vi "RandomNumPan.vi"(8 "error in (no error)":errorcluster caption="entrée d'erreur (pas d'erreur)", 11 "Tools.lvclass":refnum<class "Tools.lvclass">) -> (0 "error out":errorcluster caption="sortie d'erreur", 3 "Tools.lvclass Out":refnum<class "Tools.lvclass">)   [LabVIEW 2019, in "Tools.lvclass"]
uses:
  Tools.lvclass
  C:/Programmes Labview/LabScanV1A/DevicesClass/BaseDevice/BaseDevice.lvclass
  BaseDevice/Accessor/GetClassEvent.vi
panel:
  in  "Acq":bool
  in  "MainProgQ":refnum<queue>
  in  "MainProgQEvent":refnum<user-event>
  out "MultiplierOut":dbl=1.0
  out "OffsetOut":dbl
  out "Random Number":dbl
  in  "Multiplier":dbl=1.0
  in  "Offset":dbl
  in  "Stop":bool
  in  "MiseAJour":bool
  out "Init Program":bool
  # "Out = Random Number(0-1) x Mult. +Offset"
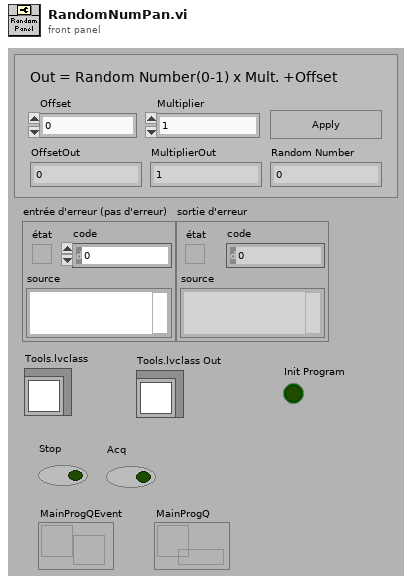
[diagram p1: front panel]
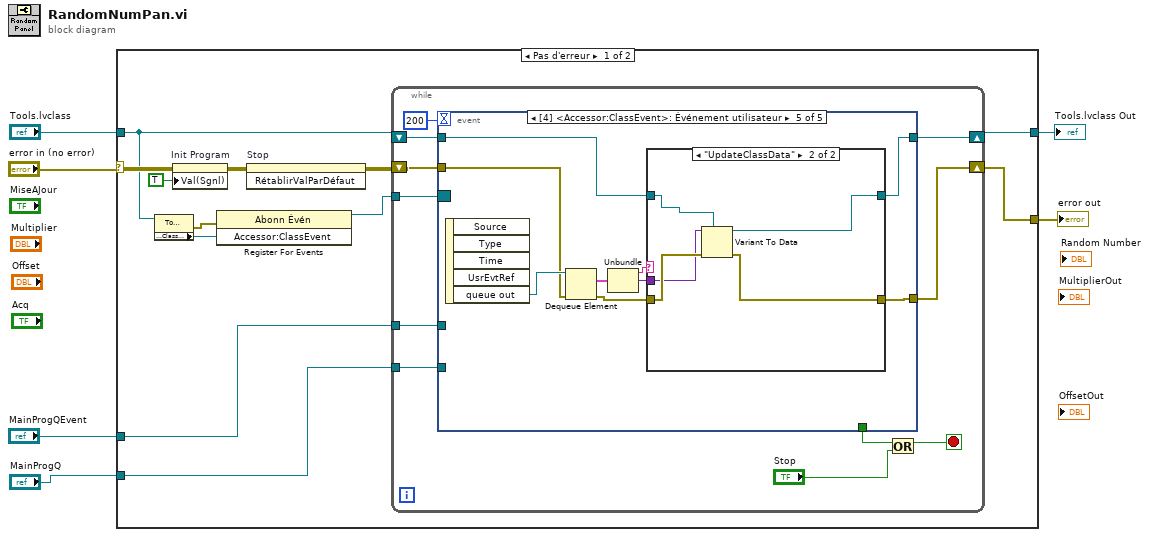
[diagram p0: block diagram]
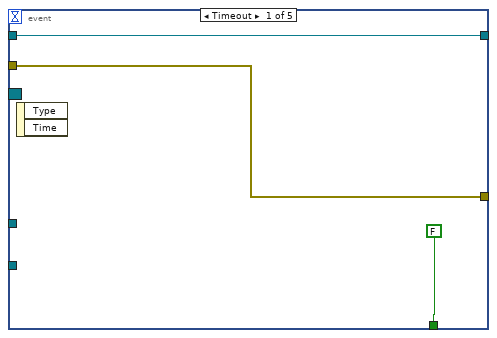
[diagram p2: hidden frame]
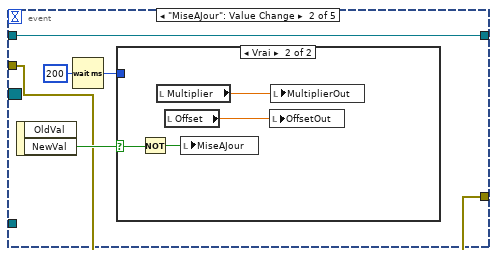
[diagram p3: hidden frame]
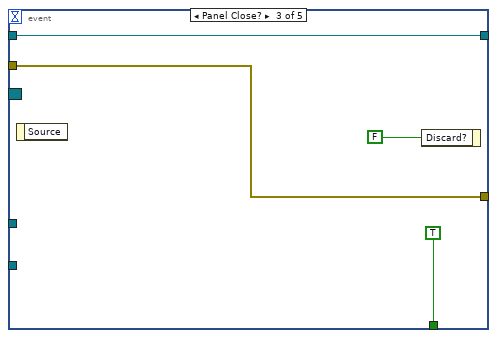
[diagram p5: hidden frame]
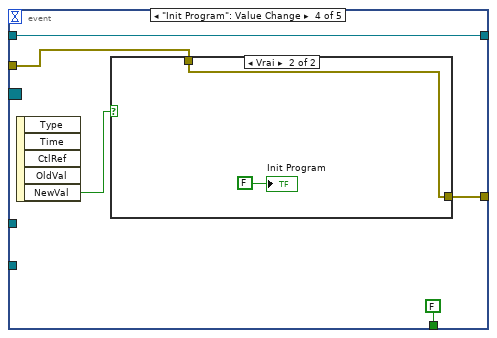
[diagram p6: hidden frame]
diagram:
  n1 = case shown="Pas d'erreur" "error in (no error)" {
    selector: "error in (no error)" -> [w15 w71]
    tunnel: [w18 w71] -> w5
    tunnel: "Tools.lvclass" -> [w8 w70]
    tunnel: [w16 w70] -> w3
    tunnel: "MainProgQEvent" -> [w12 _]
    tunnel: "MainProgQ" -> [w11 _]
    frame No Error {
      n2 = property class="Tools.lvclass"(reference=w8) -> (error out=w10:errorcluster, "Accessor:ClassEvent"=w9:refnum<user-event>)  [unwired: 1 in, 1 out]
      n3 = property on="Init Program" class="Bool (strict)"(error in=w15, "Val(Sgnl)"=TRUE ("Valeur (Signalisation)")) -> (error out=w14:errorcluster)  [unwired: 1 in, 1 out]
      n4 = register-events(error in=w10, w9) -> (reference out=w7:refnum<event-registration>)  [unwired: 1 in, 1 out]
      n5 = invoke on="Stop" class="Bool (strict)" method="RétablirValParDéfaut"(error in=w14) -> (error out=w13:errorcluster)  [unwired: 2 in, 2 out]
      n6 = while {
        shift-right: [w27] -> w18
        shift-left: w13 -> [w28]
        shift-right: [w24] -> w16
        shift-left: w8 -> [w26]
        tunnel: w12 -> [w21]
        tunnel: w11 -> [w20]
        tunnel: w7 -> [w19]
        stop <- w23 stop-if-true
        n7 = event shown="[4] <Accessor:ClassEvent>: Événement utilisateur" {
          selector: w19 -> [_ _ _ _ _]
          dyn-events: _ -> [_ _ _ _ _]
          timeout: 200 -> [_ _ _ _ _]
          tunnel: w28 -> [w30 w33 w43 w49 w60]
          tunnel: [w30 w33 w43 w48 w56] -> w27
          tunnel: w26 -> [w31 w34 w42 w47 w59]
          tunnel: [FALSE _ TRUE FALSE _] -> w25
          tunnel: [w31 w34 w42 w47 w58] -> w24
          tunnel: w21 -> [_ _ _ _ _]
          tunnel: w20 -> [_ _ _ _ _]
          event Timeout {
            n8 = event-data() -> ()  [unwired: 1 in, 2 out]
          }
          event "MiseAJour": Value Change {
            n9 = event-data() -> ("NewVal"=w37:bool)  [unwired: 1 in, 1 out]
            n10 = Wait (ms)(milliseconds to wait=u32 200 ("attente (ms)")) -> (millisecond timer value=w36:u32)
            n11 = case shown="Vrai" w37 {
              selector: w37 -> [_ w41]
              tunnel: w36 -> [_ _]
              frame False {
              }
              frame True {
                n12 = Not(x=w41) -> (.not. x?=w40:bool)
                n13 = local read "Multiplier"() -> (w39:dbl)
                n14 = local read "Offset"() -> (w38:dbl)
                n15 = local write "MiseAJour"(w40) -> ()
                n16 = local write "OffsetOut"(w38) -> ()
                n17 = local write "MultiplierOut"(w39) -> ()
              }
            }
          }
          event Panel Close? {
            n18 = event-data() -> ()  [unwired: 1 in, 1 out]
            n19 = event-data("Discard?"=FALSE ("Rejeter ?")) -> ()  [unwired: 1 in, 1 out]
          }
          event "Init Program": Value Change {
            n20 = event-data() -> ("NewVal"=w50:bool)  [unwired: 1 in, 4 out]
            n21 = case shown="Vrai" w50 {
              tunnel: w49 -> [w51 w52]
              tunnel: [w51 w52] -> w48
              frame False {
              }
              frame True {
                "Init Program" <- FALSE
              }
            }
          }
          event User Event {
            n22 = event-data() -> ("queue out"=w61:refnum<queue>)  [unwired: 1 in, 4 out]
            n23 = Dequeue Element(queue=w61, error in (no error)=w60) -> (element=w62:cluster{"Message":string, "Data":variant, i32}, error out=w55:errorcluster)  [unwired: 1 in, 2 out]
            n24 = Unbundle(w62) -> ("Message"=w57:string, "Data"=w54:variant)  [unwired: 1 out]
            n25 = case shown="\"UpdateClassData\"" w57 {
              tunnel: w59 -> [w64 w65]
              tunnel: [w64 w66] -> w58
              tunnel: [w63 w68] -> w56
              tunnel: w55 -> [w63 w69]
              tunnel: w54 -> [_ w67]
              frame Default {
              }
              frame "UpdateClassData" {
                n26 = Variant To Data(error in=w69, type=w65, Variant=w67) -> (data=w66:refnum<class "Tools.lvclass">, error out=w68:errorcluster)
              }
            }
          }
        }
        n27 = Or(x=w25, y="Stop") -> (x .or. y?=w23:bool)
      }
    }
    frame Error {
    }
  }
  "error out" <- w5
  "Tools.lvclass Out" <- w3
